vi "receive.vi"(8 "error in (no error)":errorcluster, 11 "ILCCommunications in":refnum<class "ILCCommunications.lvclass">) -> (0 "error out":errorcluster, 3 "ILCCommunications out":refnum<class "ILCCommunications.lvclass">)   [LabVIEW 2016, in "ILCCommunications.lvclass"]
uses:
  ILCCommunications.lvclass
  Common_RT_Modbus/DynamicFrameParser/DynamicFrameParser.lvclass
  ILCCommunications.lvclass/ILCCommunications.ctl
  Common_RT_Modbus/IModbus/IModbus.lvclass
  Common_RT_FPGA/IReadU16FIFO/IReadU16FIFO.lvclass
  Common_RT_HPILC/HPILC/HPILC.lvclass
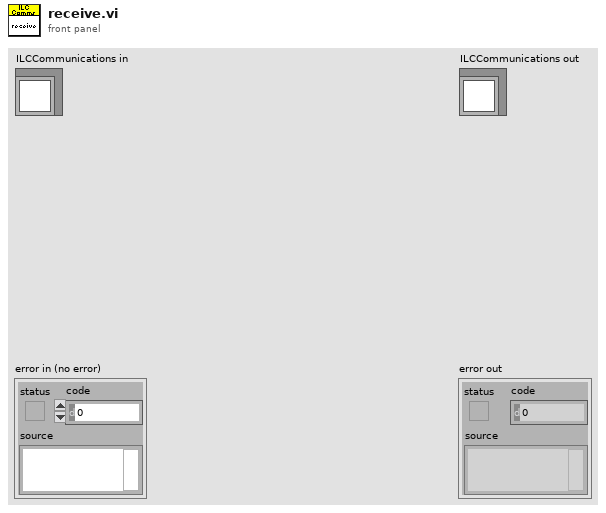
[diagram p1: front panel]
types:
  T1 = typedef "RTModbus.lvlib/RxFrame.ctl" = cluster{"Data":u8[], "Timestamp":u64}
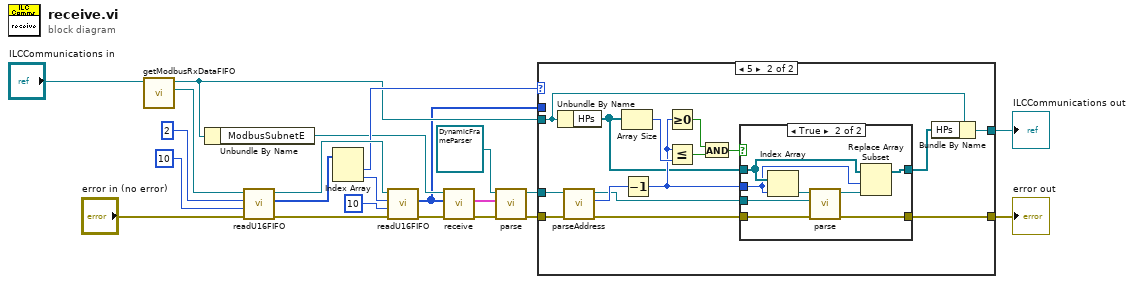
[diagram p0: block diagram]
diagram:
  n1 = call "getModbusRxDataFIFO.vi"("ILCCommunications in"="ILCCommunications in") -> ("ModbusRxDataFIFO"=w21:refnum<class "IReadU16FIFO.lvclass">, "ILCCommunications out"=w13:refnum<class "ILCCommunications.lvclass">)  [unwired: 9 in]
  n2 = Unbundle By Name(w13) -> ("ModbusSubnetE"=w12:refnum<class "IModbus.lvclass">)
  n3 = call-dynamic "readU16FIFO.vi"("error in (no error)"="error in (no error)", "Timeout"=10, "NumberOfElements"=u32 2, "IReadU16FIFO in"=w21) -> ("error out"=w5:errorcluster, "Data"=w18:u16[], "IReadU16FIFO out"=w17:refnum<class "IReadU16FIFO.lvclass">)  [unwired: 4 in, 1 out]
  n4 = Index Array(array=w18) -> (element #1=w14:u16, element #2=w16:u16)  [unwired: 2 in]
  n5 = call-dynamic "readU16FIFO.vi"("error in (no error)"=w5, "Timeout"=10, "NumberOfElements"=w16, "IReadU16FIFO in"=w17) -> ("error out"=w4:errorcluster, "Data"=w11:u16[])  [unwired: 4 in, 2 out]
  n6 = call-dynamic "receive.vi"("error in (no error)"=w4, "Data"=w11, "IModbus in"=w12) -> ("error out"=w3:errorcluster, "RxFrame"=w9:T1)  [unwired: 6 in, 1 out]
  n7 = call "parse.vi"("error in (no error)"=w3, "RxFrame"=w9, "FrameParser in"=refnum<class "DynamicFrameParser.lvclass"> refnum ("RTModbus.lvlib:DynamicFrameParser.lvclass")) -> ("error out"=w2:errorcluster, "FrameParser out"=w8:refnum<class "DynamicFrameParser.lvclass">)  [unwired: 7 in]
  n8 = case shown="5" w14 {
    tunnel: w13 -> [w24 w30]
    tunnel: w11 -> [_ _]
    tunnel: w8 -> [_ w34]
    tunnel: [w24 w28] -> w7
    tunnel: w2 -> [w23 w27]
    tunnel: [w23 w25] -> w1
    frame 0, Default {
    }
    frame 5 {
      n9 = Unbundle By Name(w30) -> ("HPs"=w32:refnum<class "HPILC.lvclass">[])
      n10 = call "parseAddress.vi"("error in (no error)"=w27, "FrameParser in"=w34) -> ("error out"=w26:errorcluster, "Address"=w33:u8, "FrameParser out"=w31:refnum<class "DynamicFrameParser.lvclass">)  [unwired: 7 in]
      n11 = Array Size(array=w32) -> (size(s)=w37:i32)
      n12 = Decrement(x=w33) -> (x-1=w35:u8)
      n13 = Greater Or Equal To 0?(x=w35) -> (x >= 0?=w39:bool)
      n14 = Less Or Equal?(x=w35, y=w37) -> (x <= y?=w38:bool)
      n15 = And(x=w39, y=w38) -> (x .and. y?=w36:bool)
      n16 = case shown="True" w36 {
        tunnel: w35 -> [_ w46]
        tunnel: w32 -> [w41 w47]
        tunnel: w31 -> [_ w48]
        tunnel: [w41 w44] -> w29
        tunnel: w26 -> [w40 w43]
        tunnel: [w40 w42] -> w25
        frame False {
        }
        frame True {
          n17 = Index Array(array=w47, index=w46) -> (element=w49:refnum<class "HPILC.lvclass">)
          n18 = call-dynamic "parse.vi"("error in (no error)"=w43, "DynamicFrameParser"=w48, "HPILC in"=w49) -> ("error out"=w42:errorcluster, "HPILC out"=w45:refnum<class "HPILC.lvclass">)  [unwired: 6 in, 1 out]
          n19 = Replace Array Subset(array=w47, new element=w45, index=w46) -> (w44:refnum<class "HPILC.lvclass">[])
        }
      }
      n20 = Bundle By Name(cluster=w30, "HPs"=w29) -> (w28:refnum<class "ILCCommunications.lvclass">)
    }
  }
  "error out" <- w1
  "ILCCommunications out" <- w7
